vi "test_3458.vi"() -> ()   [LabVIEW 2020, in "3458A Virtual Digitizer.lvlib"]
uses:
  3458A Virtual Digitizer.lvlib
  3458A Digitizer Session.ctl
  3458A Virtual Channel Config.ctl
  Counter/Counter Session.ctl
  Counter/Counter Type.ctl
  AWG/AWG Session.ctl
  AWG/AWG Type.ctl
  AWG/CMI Clock Divider v2/CMI ckd2 Session.ctl
  AWG/CMI Clock Divider v2/CMI ckd2 Source Mode.ctl
  3458A Sync Mode.ctl
  3458A Idn Mode.ctl
  3458A Digitizing Low Levels/Configure/Sampling Mode.ctl
  3458A Digitizing Process Options.ctl
  3458A Data Packet.ctl
  3458A Aux Record Data.ctl
  3458A Digitizing Low Levels/Configure/Level Setup.ctl
  3458A Digitizing Low Levels/Configure/First Sample Trigger.ctl
  3458A Aperture Selection Mode.ctl
  3458A Multiplexing Config.ctl
  Fluke 8588A/F8588A Low Pass Filter.ctl
  Fluke 8588A/F8588A Phase Lock.ctl
  Fluke 8588A/F8588A Coupling.ctl
  Counter/Counter.lvlib
  AWG/AWG.lvlib
  3458A Digitizing Low Levels/3458A Digitizing Low Levels.lvlib
panel:
  in  "TRIG source (AUTO)":T1
  out "aux data out":T2={"channel id"=0, "valid?"=[], "gain [V]"=[], "timestamp [s]"=[], "Ts [s]"=0.0, "abs timestamp"=timestamp(0 s since 1904-01-01), "t [deg C]"=[], "multiplex timestamp [s]"=-1.0, "only multiplex?"=FALSE, "multiplex smpl offset"=0, "overflow?"=FALSE}
  out "sync unit idn string":string
  out "dmm(s) idn strings":string[](array[string])
  in  "awg unit.type":T3
  in  "awg unit.VISA":refnum<visa-resource-name>
  in  "sync unit.type":T4
  in  "sync unit.VISA":refnum<visa-resource-name>
  in  "apperture [s] (1.4us)":dbl=1.4e-06 format="%#_6p"
  in  "sampling mode":T5
  in  "sync mode":T6
  in  "btn stop":bool
  out "offset [smpl]":i32
  in  "decimate by":i32=10000
  out "sampling?":bool
  out "queue buffer [%]":dbl format="%1.1f"
  in  "use streaming":bool
  in  "channels":T7[](array[typedef]) {"Range [Vpk]" min=0.0}
  out "card buffer [%]":dbl format="%1.1f"
  out "size(s)":i32[](array[numeric])
  out "Waveform Graph":dbl[][](graph)
  in  "samples count":i32=50000 min=1 format="%.0p"
  in  "fs [Hz]":dbl=50000.0 format="%#_6p"
  out "error out":errorcluster
  out "combined idn string":string
  in  "btn start":bool
  in  "dmms":T8={"channels"=[], "sync unit"={"VISA"="", "type"=enum."Picotest U6200A"}, "awg unit"={"type"=enum."Agilent 331xxA to 332xxA", "VISA"="", "enable 10MHz ref"=FALSE, "cmi ckd2"={"VISA"="", "clock source"=enum."Auto", "manual ref clk"=FALSE, "ref clock [Hz]"=0.0}}, "sync mode"=enum."MASTER-SLAVE, MASTER clocked by TIMER", "streaming mode"=FALSE, "idn mode"=enum."Auto", "sampling mode"=enum."DCV", "Ts [s]"=0.0, "sample memory [B]"=0, "proc setup"={"channel id"=0, "packet size [smpl]"=0, "current timeout [s]"=0.0, "blk2blk timeout [s]"=0.0, "event time"=timestamp(0 s since 1904-01-01), "stop notifier"=refnum, "data queues"=[], "proc refs"=[], "bus semaphore"=refnum}, "sample size [B]"=0, "sample count"=0, "aux data"={"channel id"=0, "valid?"=[], "gain [V]"=[], "timestamp [s]"=[], "Ts [s]"=0.0, "abs timestamp"=timestamp(0 s since 1904-01-01), "t [deg C]"=[], "multiplex timestamp [s]"=-1.0, "only multiplex?"=FALSE, "multiplex smpl offset"=0, "overflow?"=FALSE}, "ranges [V]"=[], "aperture [s]"=0.0, "LEVEL trigger"={"edge"=enum."POS", "level [V]"=0.0, "coupling"=enum."DC"}, "trigger mode"=enum."AUTO", "measure temp.?"=FALSE, "disp mesages"=[], "shared bus?"=FALSE, "disable display?"=FALSE, "aper mode"=enum."Manual", "aper rules"=[], "multiplex"={"cycles"=0, "delay [s]"=0.0, "enabled"=FALSE, "overhead [s]"=1.0, "tot smpls"=0, "sub-rec"=0, "overhead [%]"=0.0}, "F8588 lpf"=enum."Off", "F8588 pll"=enum."Off", "F8588 couple"=enum."DC, auto"} {"channels"."Range [Vpk]" min=0.0}
  in  "btn exit":bool
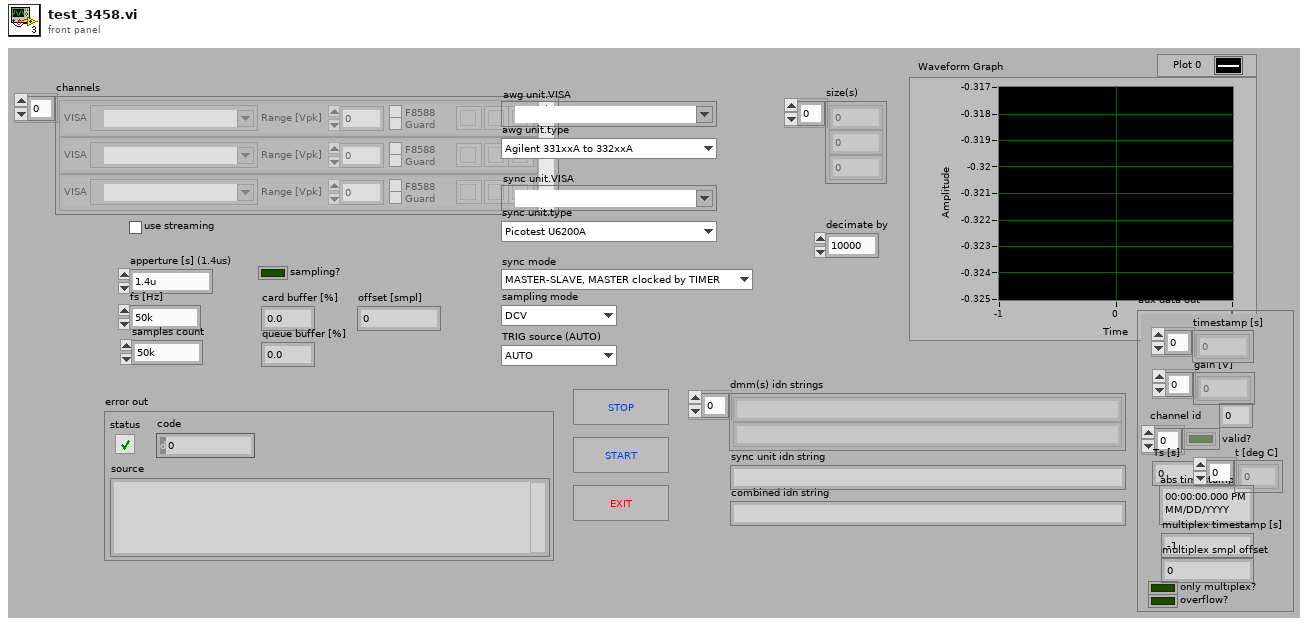
[diagram p1: front panel]
types:
  T1 = typedef "3458A Virtual Digitizer.lvlib/3458A Digitizing Low Levels.lvlib/First Sample Trigger.ctl" = enum16{"AUTO", "EXT", "SYN", "SGL", "HOLD", "LEVEL"}
  T2 = typedef "3458A Virtual Digitizer.lvlib/3458A Aux Record Data.ctl" = cluster{"channel id":i32, "valid?":bool[], "gain [V]":dbl[], "timestamp [s]":dbl[], "Ts [s]":dbl, "abs timestamp":timestamp, "t [deg C]":dbl[], "multiplex timestamp [s]":dbl, "only multiplex?":bool, "multiplex smpl offset":i64, "overflow?":bool}
  T3 = typedef "AWG.lvlib/AWG Type.ctl" = enum16{"Agilent 331xxA to 332xxA", "Agilent 335xxA to 336xxA", "Tektronix AFG3101C", "CMI Clock Divider v2", "dummy"}
  T4 = typedef "Counter.lvlib/Counter Type.ctl" = enum16{"Picotest U6200A", "dummy"}
  T5 = typedef "3458A Virtual Digitizer.lvlib/3458A Digitizing Low Levels.lvlib/Sampling Mode.ctl" = enum16{"DCV", "DSDC", "DSAC"}
  T6 = typedef "3458A Virtual Digitizer.lvlib/3458A Sync Mode.ctl" = enum16{"MASTER-SLAVE, MASTER clocked by TIMER", "MASTER-SLAVE, MASTER clocked by AWG", "ALL clocked by AWG", "MASTER-SLAVE, ALL clocked by TIMER", "ALL clocked by AWG with DFLL"}
  T7 = typedef "3458A Virtual Digitizer.lvlib/3458A Virtual Channel Config.ctl" = cluster{"VISA":refnum<visa-resource-name>, "Range [Vpk]":dbl, "btn clr":bool, "btn up":bool, "btn down":bool, "F8588":bool, "F8588 guard":bool}
  T8 = typedef "3458A Virtual Digitizer.lvlib/3458A Digitizer Session.ctl" = cluster{"channels":T7[], "sync unit":T9, "awg unit":T10, "sync mode":T6, "streaming mode":bool, "idn mode":T13, "sampling mode":T5, "Ts [s]":dbl, "sample memory [B]":i32, "proc setup":T14, "sample size [B]":i32, "sample count":i32, "aux data":T2, "ranges [V]":dbl[], "aperture [s]":dbl, "LEVEL trigger":T16, "trigger mode":T1, "measure temp.?":bool, "disp mesages":string[], "shared bus?":bool, "disable display?":bool, "aper mode":T17, "aper rules":dbl[][], "multiplex":T18, "F8588 lpf":T19, "F8588 pll":T20, "F8588 couple":T21}
  T9 = typedef "Counter.lvlib/Counter Session.ctl" = cluster{"VISA":refnum<visa-resource-name>, "type":T4}
  T10 = typedef "AWG.lvlib/AWG Session.ctl" = cluster{"type":T3, "VISA":refnum<visa-resource-name>, "enable 10MHz ref":bool, "cmi ckd2":T11}
  T11 = typedef "AWG.lvlib/CMI ckd2 Session.ctl" = cluster{"VISA":refnum<visa-resource-name>, "clock source":T12, "manual ref clk":bool, "ref clock [Hz]":dbl}
  T12 = typedef "AWG.lvlib/CMI ckd2 Source Mode.ctl" = enum16{"Auto", "LF clock", "HF clock", "Internal"}
  T13 = typedef "3458A Virtual Digitizer.lvlib/3458A Idn Mode.ctl" = enum16{"Auto", "Sequential (chn A, chn B, ...)", "From calibration string"}
  T14 = typedef "3458A Virtual Digitizer.lvlib/3458A Digitizing Process Options.ctl" = cluster{"channel id":i32, "packet size [smpl]":i32, "current timeout [s]":dbl, "blk2blk timeout [s]":dbl, "event time":timestamp, "stop notifier":refnum<notifier>, "data queues":refnum<queue>[], "proc refs":refnum<vi>[], "bus semaphore":T15}
  T15 = typedef "Semaphore RefNum" = refnum<k1>
  T16 = typedef "3458A Virtual Digitizer.lvlib/3458A Digitizing Low Levels.lvlib/Level Setup.ctl" = cluster{"edge":enum16{"POS", "NEG"}, "level [V]":dbl, "coupling":enum16{"DC", "AC"}}
  T17 = typedef "3458A Virtual Digitizer.lvlib/3458A Aperture Selection Mode.ctl" = enum16{"Manual", "Maximum", "Table"}
  T18 = typedef "3458A Multiplexing Config.ctl" = cluster{"cycles":i32, "delay [s]":dbl, "enabled":bool, "overhead [s]":dbl, "tot smpls":i64, "sub-rec":i32, "overhead [%]":dbl}
  T19 = typedef "F8588A Low Pass Filter.ctl" = enum16{"Off", "100 kHz", "3 MHz"}
  T20 = typedef "F8588A Phase Lock.ctl" = enum16{"Off", "1 MHz", "10 MHz"}
  T21 = typedef "F8588A Coupling.ctl" = enum16{"AC, 1 MOhm", "AC, 10 MOhm", "DC, 1 MOhm", "DC, 10 MOhm", "DC, auto"}
  T22 = typedef "3458A Virtual Digitizer.lvlib/3458A Data Packet.ctl" = cluster{"data":i32[][], "offset [smpl]":i32, "count [smpl]":i32, "all done?":bool, "sampling?":bool, "queue buffer [%]":dbl, "valid?":bool, "overflow?":bool}
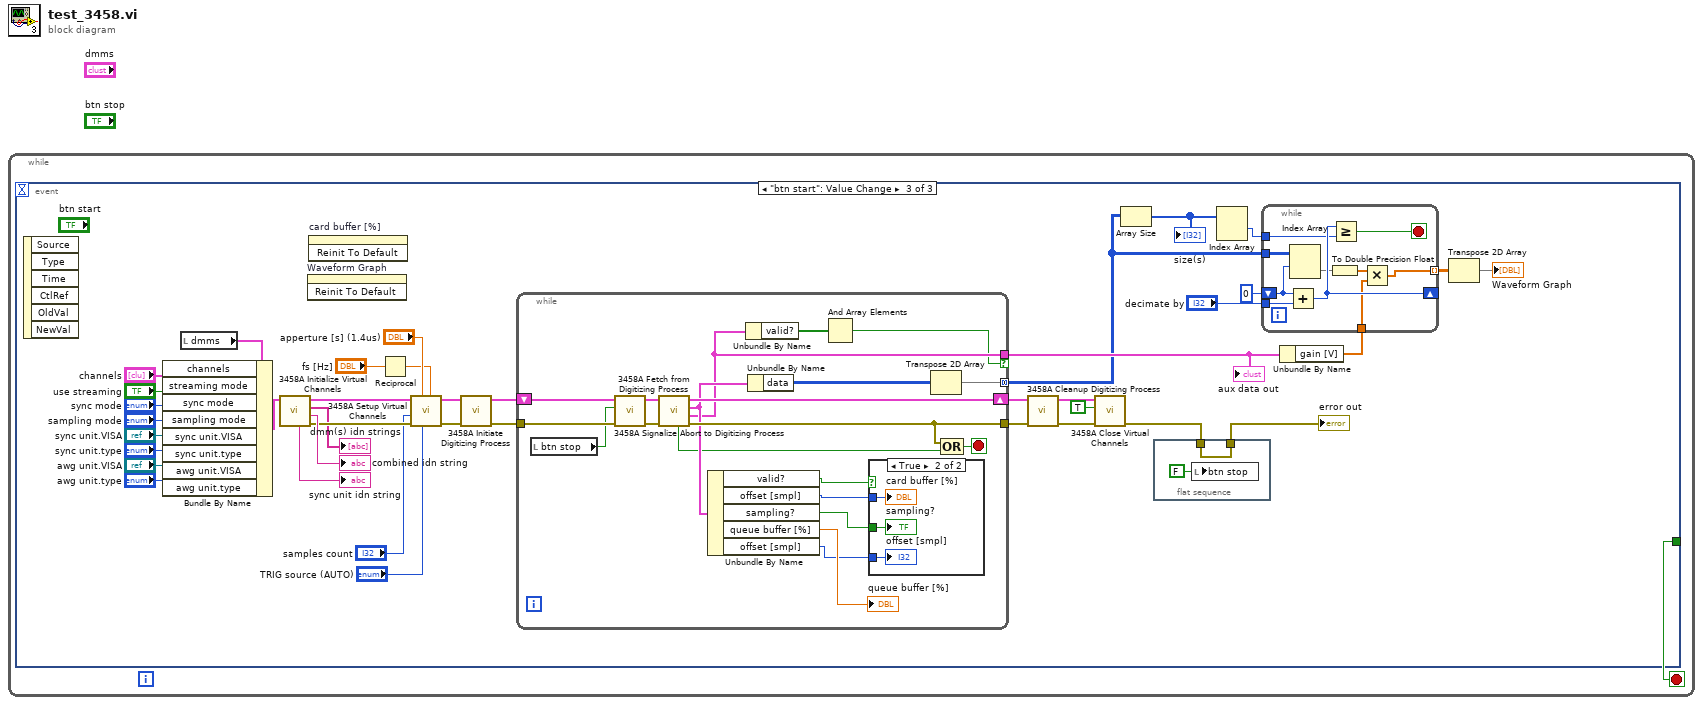
[diagram p0: block diagram]
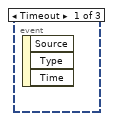
[diagram p2: hidden frame]
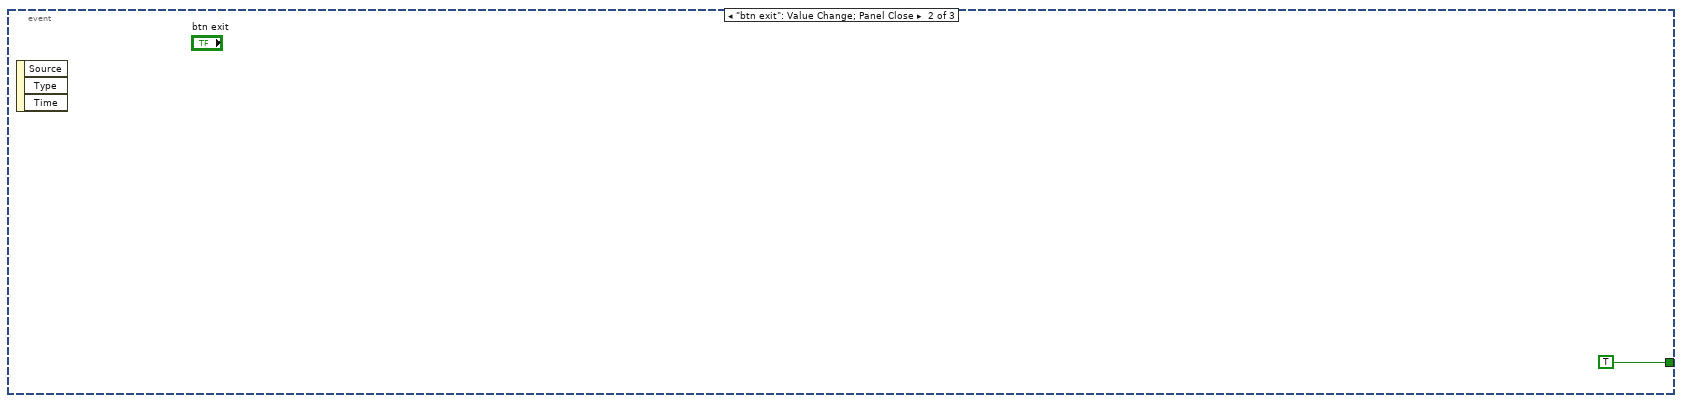
[diagram p3: hidden frame]
diagram:
  n1 = while {
    stop <- w1 stop-if-true
    n2 = event shown="[2] \"btn start\": Value Change" {
      selector: _ -> [_ _ _]
      dyn-events: _ -> [_ _ _]
      timeout: _ -> [_ _ _]
      tunnel: [_ TRUE _] -> w1
      event Timeout {
        n3 = event-data() -> ()  [unwired: 1 in, 3 out]
      }
      event "btn exit": Value Change; Panel Close {
        n4 = event-data() -> ()  [unwired: 1 in, 3 out]
      }
      event "btn start": Value Change {
        n5 = event-data() -> ()  [unwired: 1 in, 6 out]
        n6 = local read "dmms"() -> (w30:T8)
        n7 = Bundle By Name(cluster=w30, "channels"="channels", "streaming mode"="use streaming", "sync mode"="sync mode", "sampling mode"="sampling mode", "sync unit.VISA"="sync unit.VISA", "sync unit.type"="sync unit.type", "awg unit.VISA"="awg unit.VISA", "awg unit.type"="awg unit.type") -> (w11:T8)
        n8 = call "3458A Initialize Virtual Channels.vi"("digitizer in"=w11) -> ("error out"=w41:errorcluster, "awg idn string"=→"combined idn string":string, "dmm(s) idn strings"=→"dmm(s) idn strings":string[], "digitizer out"=w21:T8, "sync unit idn string"=→"sync unit idn string":string)  [unwired: 6 in]
        n9 = invoke on="Waveform Graph" class="WFGraph (strict)" method="Reinit To Default"() -> ()  [unwired: 3 in, 3 out]
        n10 = invoke on="card buffer [%]" class="DigNum (strict)" method="Reinit To Default"() -> ()  [unwired: 3 in, 3 out]
        n11 = Reciprocal(x="fs [Hz]") -> (1/x=w8:dbl)
        n12 = call "3458A Setup Virtual Channels.vi"("sample period [s] (1 ms)"=w8, "TRIG source (AUTO)"="TRIG source (AUTO)", "apperture [s] (1.4 us)"="apperture [s] (1.4us)", "error in"=w41, "samples count (100)"="samples count", "digitizer in"=w21) -> ("error out"=w39:errorcluster, "digitizer out"=w20:T8)  [unwired: 4 in]
        n13 = call "3458A Initiate Digitizing Process.vi"("error in"=w39, "session in"=w20) -> ("error out"=w38:errorcluster, "session out"=w36:T8)  [unwired: 7 in, 1 out]
        n14 = while {
          tunnel: w38 -> [w54]
          tunnel: [w63] -> w6
          tunnel: [w60] -> w24 mode=concatenating
          tunnel: [w48] -> w27 if=w46
          shift-right: [w64] -> w17
          shift-left: w36 -> [w51]
          stop <- w62 stop-if-true
          n15 = local read "btn stop"() -> (w52:bool)
          n16 = call "3458A Signalize Abort to Digitizing Process.vi"("error in"=w54, "send abort signal? (True)"=w52, "session in"=w51) -> ("error out (copy)"=w53:errorcluster, "session out"=w50:T8)  [unwired: 7 in]
          n17 = call "3458A Fetch from Digitizing Process.vi"("error in"=w53, "session in"=w50) -> ("error out"=w63:errorcluster, "aux data"=w48:T2, "data packet"=w56:T22, "session out"=w64:T8, "fetching done?"=w49:bool)  [unwired: 5 in]
          n18 = Unbundle By Name(w56) -> ("valid?"=w45:bool, "offset [smpl]"=w59:i32, "sampling?"=w57:bool, "queue buffer [%]"=→"queue buffer [%]":dbl, "offset [smpl]"=w55:i32)
          n19 = Unbundle By Name(w48) -> ("valid?"=w47:bool[])
          n20 = Unbundle By Name(w56) -> ("data"=w61:i32[][])
          n21 = And Array Elements(Boolean array=w47) -> (logical AND=w46:bool)
          n22 = case shown="True" w45 {
            tunnel: w59 -> [_ w67]
            tunnel: w57 -> [_ w66]
            tunnel: w55 -> [_ w65]
            frame False {
            }
            frame True {
              "card buffer [%]" <- w67
              "sampling?" <- w66
              "offset [smpl]" <- w65
            }
          }
          n23 = Transpose 2D Array(2D array=w61) -> (transposed array=w60:i32[][])
          n24 = Compound Arithmetic op=OR(w63, w49) -> (w62:bool)
        }
        "aux data out" <- w27
        n25 = call "3458A Cleanup Digitizing Process.vi"("error in"=w6, "session in"=w17) -> ("error out"=w37:errorcluster, "session out"=w16:T8)  [unwired: 8 in]
        n26 = call "3458A Close Virtual Channels.vi"("error in"=w37, "Reset to preset mode (True)"=TRUE, "session in"=w16) -> ("error out"=w5:errorcluster)  [unwired: 7 in, 1 out]
        n27 = Array Size(array=w24) -> (size(s)=w35:i32[])
        "size(s)" <- w35
        n28 = flat-sequence {
          tunnel: [w43] -> w4
          tunnel: w5 -> [w43]
          frame #0 {
            n29 = local write "btn stop"(FALSE ("btn stop")) -> ()
          }
        }
        n30 = Index Array(array=w35) -> (element #1=w31:i32)  [unwired: 2 in, 1 out]
        n31 = Unbundle By Name(w27) -> ("gain [V]"=w26:dbl[])
        n32 = while {
          tunnel: w31 -> [w74]
          tunnel: w24 -> [w77]
          shift-right: [w75] -> _
          shift-left: 0 -> [w72]
          tunnel: [w68] -> w32 mode=indexing
          tunnel: "decimate by" -> [w76]
          tunnel: w26 -> [w69]
          stop <- w73 stop-if-true
          n33 = Add(x=w72, y=w76) -> (x+y=w75:i32)
          n34 = Index Array(array=w77, index (row)=w72) -> (element=w71:i32[])  [unwired: 1 in]
          n35 = To Double Precision Float(number=w71) -> (double precision float=w70:dbl[])
          n36 = Greater Or Equal?(x=w75, y=w74) -> (x >= y?=w73:bool)
          n37 = Multiply(x=w70, y=w69) -> (x*y=w68:dbl[])
        }
        n38 = Transpose 2D Array(2D array=w32) -> (transposed array=→"Waveform Graph":dbl[][])
        "error out" <- w4
      }
    }
  }
